vi "Init Device.vi"(8 "error in (no error)":errorcluster, 11 "Toggle 8 (niDig) in":refnum<class "Toggle 8 (niDig).lvclass">) -> (0 "error out":errorcluster, 3 "Toggle 8 (niDig) out":refnum<class "Toggle 8 (niDig).lvclass">)   [LabVIEW 2020, in "Toggle 8 (niDig).lvclass"]
uses:
  Toggle 8 (niDig).lvclass
  niDigital.lvclass
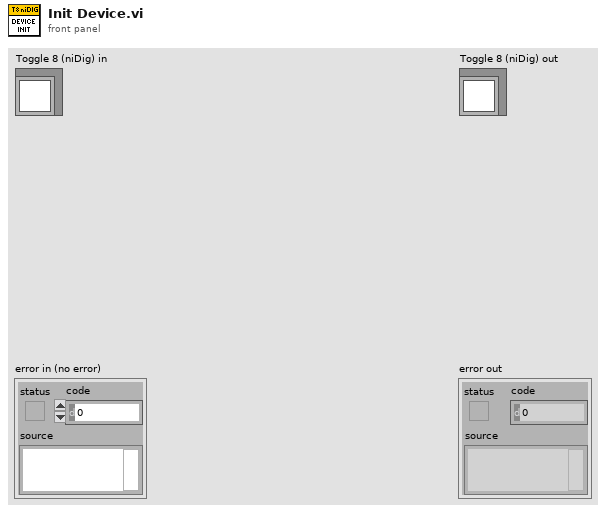
[diagram p1: front panel]
types:
  T1 = cluster{"USID":u8, "Write Address":u8, "Write Data Array":u8[]}[]
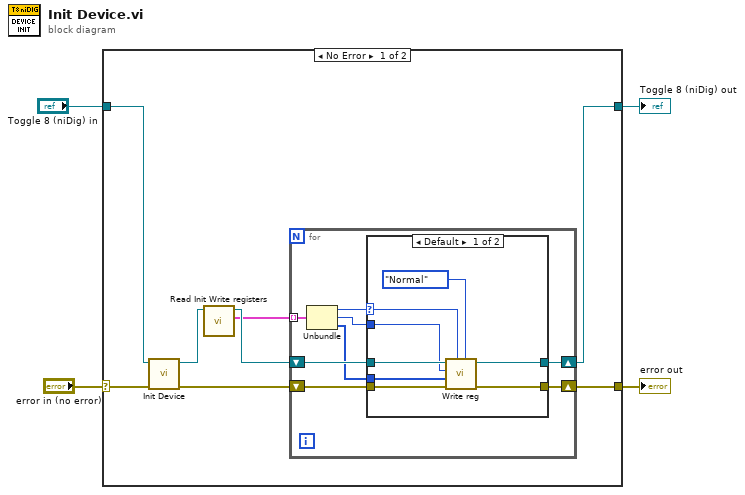
[diagram p0: block diagram]
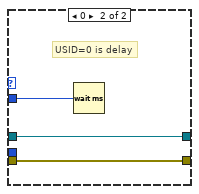
[diagram p2: hidden frame]
diagram:
  n1 = case shown="No Error" "error in (no error)" {
    selector: "error in (no error)" -> [w12 w33]
    tunnel: "Toggle 8 (niDig) in" -> [w11 w32]
    tunnel: [w7 w33] -> w2
    tunnel: [w6 w32] -> w1
    frame No Error {
      n2 = call-parent "Init Device.vi"("error in (no error)"=w12, "niDigital in"=w11) -> ("error out"=w8:errorcluster, "niDigital out"=w10:refnum<class "Toggle 8 (niDig).lvclass">)  [unwired: 8 in]
      n3 = call-dynamic "Read Init Write registers.vi"("Toggle 8 (niDig) in"=w10) -> ("Init Write registers"=w5:T1, "Toggle 8 (niDig) out"=w9:refnum<class "Toggle 8 (niDig).lvclass">)  [unwired: 9 in]
      n4 = for {
        shift-right: [w18] -> w7
        shift-left: w8 -> [w19]
        shift-right: [w17] -> w6
        shift-left: w9 -> [w20]
        tunnel: w5 -> [w16] mode=indexing
        n5 = Unbundle(w16) -> ("USID"=w15:u8, "Write Address"=w14:u8, "Write Data Array"=w13:u8[])
        n6 = case shown="Default" w15 {
          selector: w15 -> [w24 _]
          tunnel: w20 -> [w28 w30]
          tunnel: w19 -> [w27 w29]
          tunnel: [w26 w29] -> w18
          tunnel: [w25 w30] -> w17
          tunnel: w14 -> [w22 w31]
          tunnel: w13 -> [w21 _]
          frame Default {
            n7 = call-dynamic "Write reg.vi"("Write type"=enum16{"Normal", "Extended", "Extended Cycle"}."Normal", "Write USID"=w24, "error in (no error)"=w27, "Write Data"=w21, "Write Address"=w22, "niDigital in"=w28) -> ("error out"=w26:errorcluster, "niDigital out"=w25:refnum<class "Toggle 8 (niDig).lvclass">)  [unwired: 4 in]
          }
          frame 0 {
            # "USID=0 is delay"
            n8 = Wait (ms)(milliseconds to wait=w31) -> ()  [unwired: 1 out]
          }
        }
      }
    }
    frame Error {
    }
  }
  "error out" <- w2
  "Toggle 8 (niDig) out" <- w1
